vi "Set EXT.vi"(7 "Treatment of Infinity/NaN":T1, 8 "error in (no error)":errorcluster, 10 "Numeric":ext, 11 "JSON Scalar in":refnum<class "JSON Scalar.lvclass">) -> (0 "error out":errorcluster, 3 "JSON Scalar out":refnum<class "JSON Scalar.lvclass">)   [LabVIEW 2020, in "Library Commun.lvlib" / "JSON Scalar.lvclass"]
doc: "Stores a <b>Numeric</b> as a <b>JSON Scalar</b>.\n\nTreatment of Infinity, -Infinity, and Not-a-Number values of floating-point numerics:\n- <b>Default JSON:</b> write all as nulls.\n- <b>Extended:</b> use JSON strings for Infinities (\"Infinity\", \"-Infinity\"); NaN still null.\n- <b>LabVIEW extentions</b> (compatable with the LabVIEW JSON primatives): Infinity, -Infinity, NaN (not in quotes)\n\nNote that the LabVIEW extentions are not valid JSON. The Extended option <b>is</b> valid JSON, but not all JSON parsers will process strings as numeric values.\n\nMore information on http://lavag.org/topic/16217-cr-json-labview"
uses:
  JSON Scalar.lvclass
  Infinity&NaN.ctl
  support/JSON support.lvlib
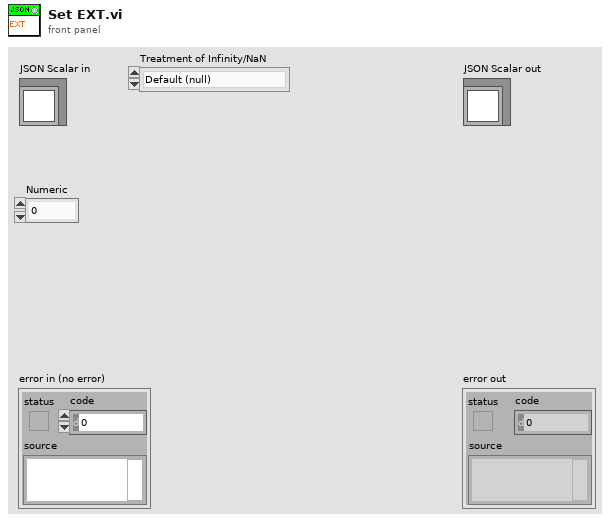
[diagram p1: front panel]
types:
  T1 = typedef "Library Commun.lvlib/JSON support.lvlib/Infinity&NaN.ctl" = enum16{"Default (null)", "Extended", "LabVIEW extensions"}
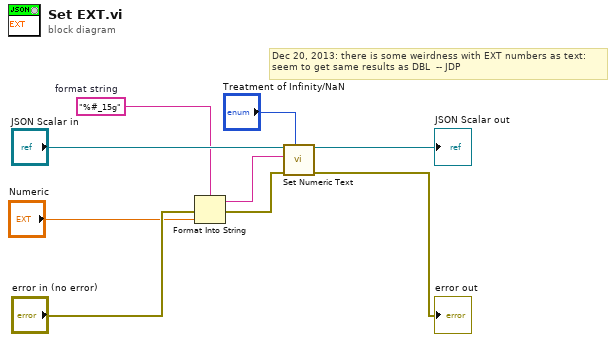
[diagram p0: block diagram]
diagram:
  w2 = "%#_15g"  # format string
  # "Dec 20, 2013: there is some weirdness with EXT numbers as text:\nseem to get same results as DBL  -- JDP"
  n1 = Format Into String(format string=w2, error in="error in (no error)", "Numeric") -> (resulting string=w4:string, error out=w3:errorcluster)  [unwired: 1 in]
  n2 = call "Set Numeric Text.vi"("Treatment of Infinity/NaN"="Treatment of Infinity/NaN", "error in (no error)"=w3, "Numeric Text"=w4, "JSON Scalar in"="JSON Scalar in") -> ("error out"=→"error out":errorcluster, "JSON Scalar out"=→"JSON Scalar out":refnum<class "JSON Scalar.lvclass">)  [unwired: 6 in]
